vi "PathPlanner_TrajectoryState_Interpolate.vi"(9 "Time":dbl, 10 "end Val":T1={"AngularAcceleration"={"VALUE"=0.0, "COS"=1.0, "SIN"=0.0}, "PositionMeters"=0.0, "TrajectoryState"={"TimeSeconds"=0.0, "Velocity"=0.0, "Acceleration"=0.0, "POSE"={"TRANSLATION"={"X"=0.0, "Y"=0.0}, "ROTATION"={"VALUE"=0.0, "COS"=1.0, "SIN"=0.0}}, "Curvature"=0.0}, "AngularVelocity"={"VALUE"=0.0, "COS"=1.0, "SIN"=0.0}, "HolonomicRotation"={"VALUE"=0.0, "COS"=1.0, "SIN"=0.0}, "CurveRadius"=0.0, "DeltaPos"=0.0} {"HolonomicRotation"."SIN" format="%13.4f"; "HolonomicRotation"."COS" format="%13.4f"; "HolonomicRotation"."VALUE" format="%13.4f"; "AngularVelocity"."SIN" format="%13.4f"; "AngularVelocity"."COS" format="%13.4f"; "AngularVelocity"."VALUE" format="%13.4f"; "TrajectoryState"."POSE"."ROTATION"."SIN" format="%13.4f"; "TrajectoryState"."POSE"."ROTATION"."COS" format="%13.4f"; "TrajectoryState"."POSE"."ROTATION"."VALUE" format="%13.4f"; "TrajectoryState"."POSE"."TRANSLATION"."Y" format="%14.3f"; "TrajectoryState"."POSE"."TRANSLATION"."X" format="%14.3f"; "AngularAcceleration"."SIN" format="%13.4f"; "AngularAcceleration"."COS" format="%13.4f"; "AngularAcceleration"."VALUE" format="%13.4f"}, 11 "in PathPlannerState":T1={"AngularAcceleration"={"VALUE"=0.0, "COS"=1.0, "SIN"=0.0}, "PositionMeters"=0.0, "TrajectoryState"={"TimeSeconds"=0.0, "Velocity"=0.0, "Acceleration"=0.0, "POSE"={"TRANSLATION"={"X"=0.0, "Y"=0.0}, "ROTATION"={"VALUE"=0.0, "COS"=1.0, "SIN"=0.0}}, "Curvature"=0.0}, "AngularVelocity"={"VALUE"=0.0, "COS"=1.0, "SIN"=0.0}, "HolonomicRotation"={"VALUE"=0.0, "COS"=1.0, "SIN"=0.0}, "CurveRadius"=0.0, "DeltaPos"=0.0} {"HolonomicRotation"."SIN" format="%13.4f"; "HolonomicRotation"."COS" format="%13.4f"; "HolonomicRotation"."VALUE" format="%13.4f"; "AngularVelocity"."SIN" format="%13.4f"; "AngularVelocity"."COS" format="%13.4f"; "AngularVelocity"."VALUE" format="%13.4f"; "TrajectoryState"."POSE"."ROTATION"."SIN" format="%13.4f"; "TrajectoryState"."POSE"."ROTATION"."COS" format="%13.4f"; "TrajectoryState"."POSE"."ROTATION"."VALUE" format="%13.4f"; "TrajectoryState"."POSE"."TRANSLATION"."Y" format="%14.3f"; "TrajectoryState"."POSE"."TRANSLATION"."X" format="%14.3f"; "AngularAcceleration"."SIN" format="%13.4f"; "AngularAcceleration"."COS" format="%13.4f"; "AngularAcceleration"."VALUE" format="%13.4f"}) -> (3 "interpolated PathPlanner State":T1={"AngularAcceleration"={"VALUE"=0.0, "COS"=1.0, "SIN"=0.0}, "PositionMeters"=0.0, "TrajectoryState"={"TimeSeconds"=0.0, "Velocity"=0.0, "Acceleration"=0.0, "POSE"={"TRANSLATION"={"X"=0.0, "Y"=0.0}, "ROTATION"={"VALUE"=0.0, "COS"=1.0, "SIN"=0.0}}, "Curvature"=0.0}, "AngularVelocity"={"VALUE"=0.0, "COS"=1.0, "SIN"=0.0}, "HolonomicRotation"={"VALUE"=0.0, "COS"=1.0, "SIN"=0.0}, "CurveRadius"=0.0, "DeltaPos"=0.0} {"HolonomicRotation"."SIN" format="%13.4f"; "HolonomicRotation"."COS" format="%13.4f"; "HolonomicRotation"."VALUE" format="%13.4f"; "AngularVelocity"."SIN" format="%13.4f"; "AngularVelocity"."COS" format="%13.4f"; "AngularVelocity"."VALUE" format="%13.4f"; "TrajectoryState"."POSE"."ROTATION"."SIN" format="%13.4f"; "TrajectoryState"."POSE"."ROTATION"."COS" format="%13.4f"; "TrajectoryState"."POSE"."ROTATION"."VALUE" format="%13.4f"; "TrajectoryState"."POSE"."TRANSLATION"."Y" format="%14.3f"; "TrajectoryState"."POSE"."TRANSLATION"."X" format="%14.3f"; "AngularAcceleration"."SIN" format="%13.4f"; "AngularAcceleration"."COS" format="%13.4f"; "AngularAcceleration"."VALUE" format="%13.4f"})   [LabVIEW 2019, in "PathPlanner.lvlib"]
uses:
  PathPlanner.lvlib
  PathPlannerState.ctl
  <vilib>/Rock Robotics/WPI/ThirdParty/JAS_Junk/TrajLib/ROTATION2D.ctl
  <vilib>/Rock Robotics/WPI/ThirdParty/JAS_Junk/TrajLib/TRAJ_STATE.ctl
  <vilib>/Rock Robotics/WPI/ThirdParty/JAS_Junk/TrajLib/POSE2D.ctl
  <vilib>/Rock Robotics/WPI/ThirdParty/JAS_Junk/TrajLib/TRANSLATION2D.ctl
  <vilib>/Rock Robotics/WPI/ThirdParty/JAS_Junk/TrajLib/Trajectory_Library.lvlib
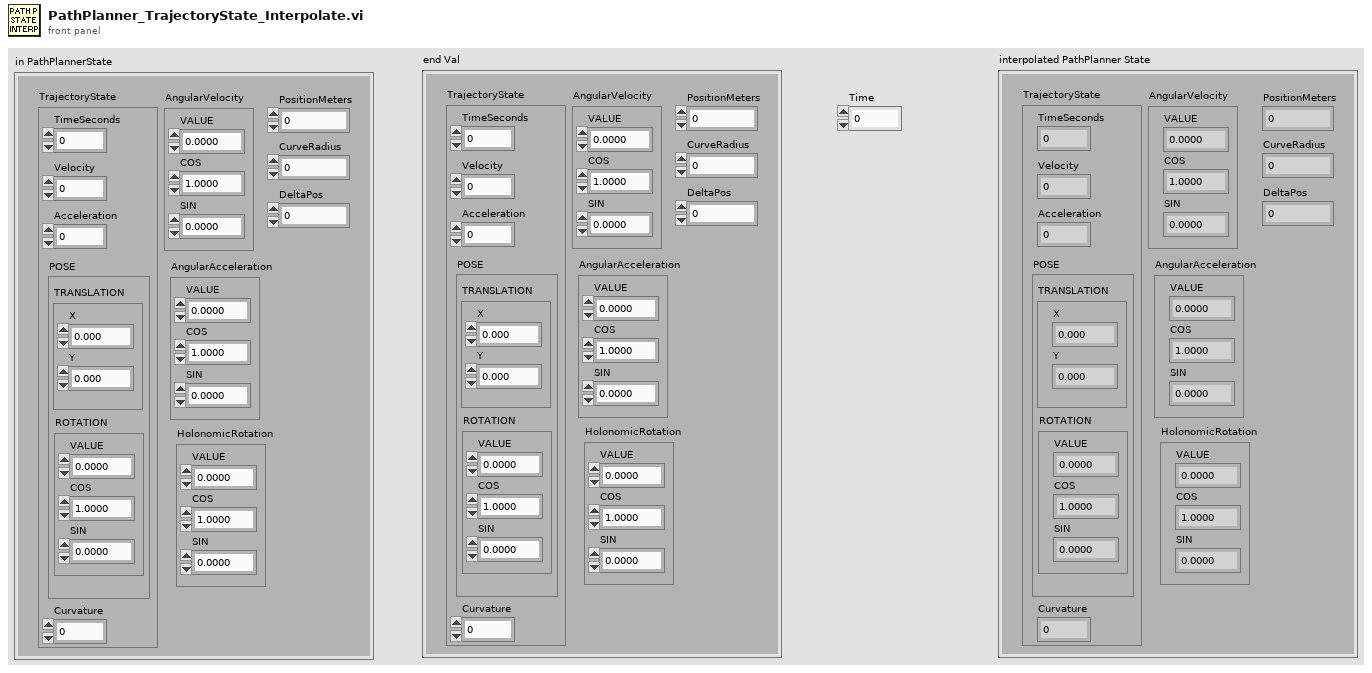
[diagram p1: front panel]
types:
  T1 = typedef "PathPlanner.lvlib/PathPlannerState.ctl" = cluster{"AngularAcceleration":T2, "PositionMeters":dbl, "TrajectoryState":T3, "AngularVelocity":T2, "HolonomicRotation":T2, "CurveRadius":dbl, "DeltaPos":dbl}
  T2 = typedef "Trajectory_Library.lvlib/ROTATION2D.ctl" = cluster{"VALUE":dbl, "COS":dbl, "SIN":dbl}
  T3 = typedef "Trajectory_Library.lvlib/TRAJ_STATE.ctl" = cluster{"TimeSeconds":dbl, "Velocity":dbl, "Acceleration":dbl, "POSE":T4, "Curvature":dbl}
  T4 = typedef "Trajectory_Library.lvlib/POSE2D.ctl" = cluster{"TRANSLATION":T5, "ROTATION":T2}
  T5 = typedef "Trajectory_Library.lvlib/TRANSLATION2D.ctl" = cluster{"X":dbl, "Y":dbl}
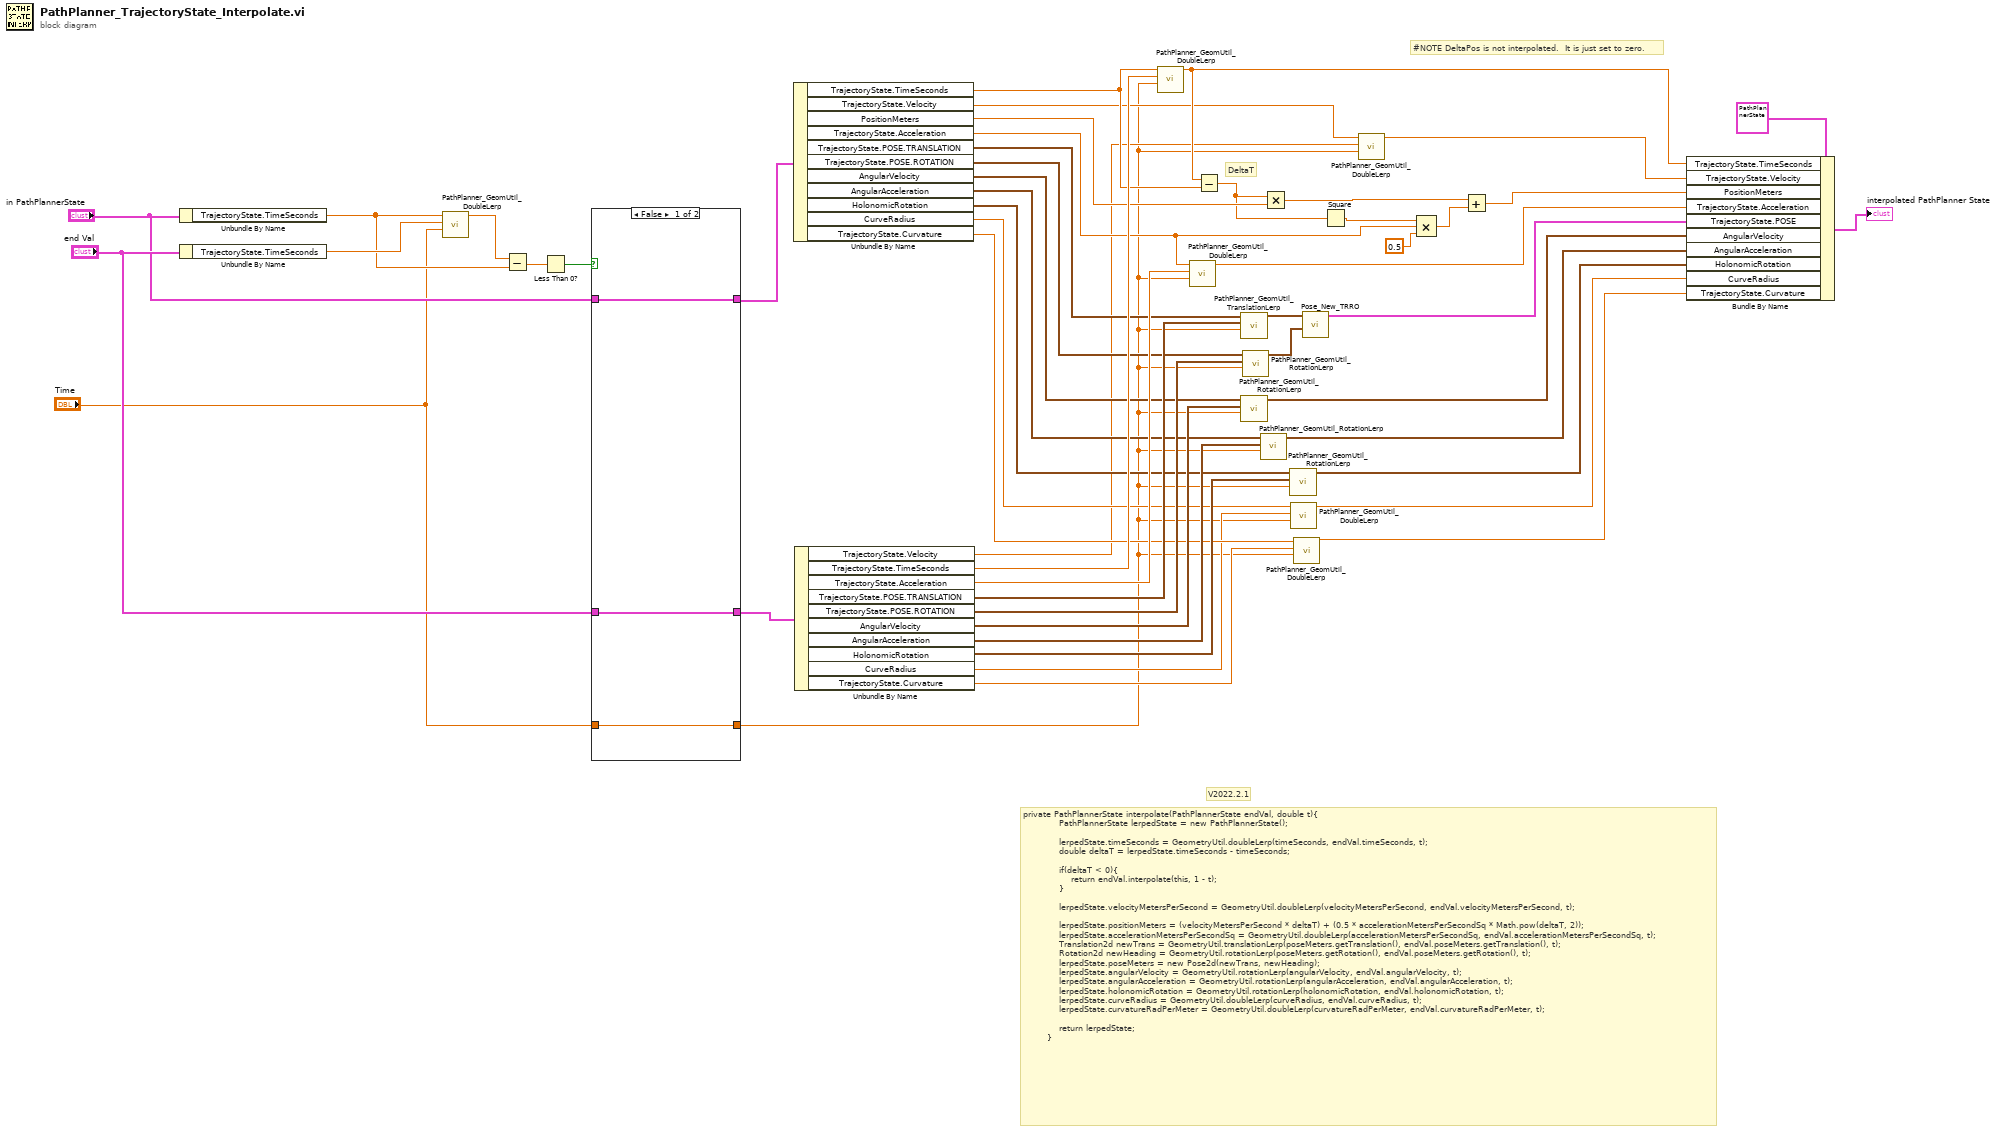
[diagram p0: block diagram]
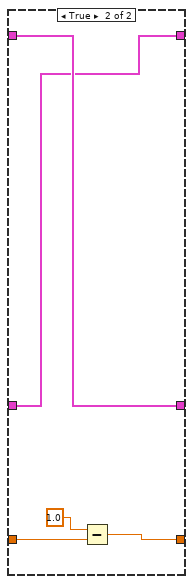
[diagram p2: hidden frame]
diagram:
  # "V2022.2.1"
  # "private PathPlannerState interpolate(PathPlannerState endVal, double t){\n            PathPlannerState lerpedState = new PathPlannerState();\n\n            lerpedState.timeSeconds = GeometryUtil.doubleLerp(timeSeconds, endVal.timeSeconds, t);\n            double deltaT = lerpedState.timeSeconds - timeSeconds;\n\n            if(deltaT < 0){\n                return endVal.interpolate(this, 1 - t);\n            }\n\n            lerpedState.velocityMetersPerSecond = GeometryUtil.doubleLerp(velocityMetersPerSecond, endVal.velocityMetersPerSecond, t);\n\n            lerpedState.positionMeters = (velocityMetersPerSecond * deltaT) + (0.5 * accelerationMetersPerSecondSq * Math.pow(deltaT, 2));\n            lerpedState.accelerationMetersPerSecondSq = GeometryUtil.doubleLerp(accelerationMetersPerSecondSq, endVal.accelerationMetersPerSecondSq, t);\n            Translation2d newTrans = GeometryUtil.translationLerp(poseMeters.getTranslation(), endVal.poseMeters.getTranslation(), t);\n            Rotation2d newHeading = GeometryUtil.rotationLerp(poseMeters.getRotation(), endVal.poseMeters.getRotation(), t);\n            lerpedState.poseMeters = new Pose2d(newTrans, newHeading);\n            lerpedState.angularVelocity = GeometryUtil.rotationLerp(angularVelocity, endVal.angularVelocity, t);\n            lerpedState.angularAcceleration = GeometryUtil.rotationLerp(angularAcceleration, endVal.angularAcceleration, t);\n            lerpedState.holonomicRotation = GeometryUtil.rotationLerp(holonomicRotation, endVal.holonomicRotation, t);\n            lerpedState.curveRadius = GeometryUtil.doubleLerp(curveRadius, endVal.curveRadius, t);\n            lerpedState.curvatureRadPerMeter = GeometryUtil.doubleLerp(curvatureRadPerMeter, endVal.curvatureRadPerMeter, t);\n\n            return lerpedState;\n        }"
  # "#NOTE DeltaPos is not interpolated.  It is just set to zero."
  # "DeltaT"
  n1 = Unbundle By Name("in PathPlannerState") -> ("TrajectoryState.TimeSeconds"=w47:dbl)
  n2 = Unbundle By Name("end Val") -> ("TrajectoryState.TimeSeconds"=w49:dbl)
  n3 = call "PathPlanner_GeomUtil_DoubleLerp.vi"("T"="Time", "EndVal"=w49, "StartVal"=w47) -> ("Lerp"=w48:dbl)  [unwired: 8 in]
  n4 = Subtract(x=w48, y=w47) -> (x-y=w46:dbl)
  n5 = Less Than 0?(x=w46) -> (x < 0?=w45:bool)
  n6 = case shown="False" w45 {
    tunnel: "end Val" -> [w54 w58]
    tunnel: [w54 w59] -> w40
    tunnel: "in PathPlannerState" -> [w53 w59]
    tunnel: [w53 w58] -> w41
    tunnel: [w52 w55] -> w1
    tunnel: "Time" -> [w52 w56]
    frame False {
    }
    frame True {
      n7 = Subtract(x=1.0, y=w56) -> (x-y=w55:dbl)
    }
  }
  n8 = Unbundle By Name(w41) -> ("TrajectoryState.TimeSeconds"=w37:dbl, "TrajectoryState.Velocity"=w3:dbl, "PositionMeters"=w36:dbl, "TrajectoryState.Acceleration"=w29:dbl, "TrajectoryState.POSE.TRANSLATION"=w26:T5, "TrajectoryState.POSE.ROTATION"=w24:T2, "AngularVelocity"=w19:T2, "AngularAcceleration"=w16:T2, "HolonomicRotation"=w13:T2, "CurveRadius"=w10:dbl, "TrajectoryState.Curvature"=w9:dbl)
  n9 = Unbundle By Name(w40) -> ("TrajectoryState.Velocity"=w2:dbl, "TrajectoryState.TimeSeconds"=w39:dbl, "TrajectoryState.Acceleration"=w28:dbl, "TrajectoryState.POSE.TRANSLATION"=w25:T5, "TrajectoryState.POSE.ROTATION"=w23:T2, "AngularVelocity"=w18:T2, "AngularAcceleration"=w15:T2, "HolonomicRotation"=w12:T2, "CurveRadius"=w8:dbl, "TrajectoryState.Curvature"=w7:dbl)
  n10 = call "PathPlanner_GeomUtil_DoubleLerp.vi"("T"=w1, "EndVal"=w39, "StartVal"=w37) -> ("Lerp"=w38:dbl)  [unwired: 8 in]
  n11 = call "PathPlanner_GeomUtil_DoubleLerp.vi"("T"=w1, "EndVal"=w28, "StartVal"=w29) -> ("Lerp"=w27:dbl)  [unwired: 8 in]
  n12 = Subtract(x=w38, y=w37) -> (x-y=w30:dbl)
  n13 = call "PathPlanner_GeomUtil_TranslationLerp.vi"("T"=w1, "EndVal"=w25, "StartVal"=w26) -> ("Lerp"=w22:T5)  [unwired: 8 in]
  n14 = call "PathPlanner_GeomUtil_RotationLerp.vi"("T"=w1, "EndVal"=w18, "StartVal"=w19) -> ("Lerp"=w17:T2)  [unwired: 8 in]
  n15 = call "PathPlanner_GeomUtil_RotationLerp.vi"("T"=w1, "EndVal"=w23, "StartVal"=w24) -> ("Lerp"=w21:T2)  [unwired: 8 in]
  n16 = call "PathPlanner_GeomUtil_RotationLerp.vi"("T"=w1, "EndVal"=w15, "StartVal"=w16) -> ("Lerp"=w14:T2)  [unwired: 8 in]
  n17 = Multiply(x=w30, y=w36) -> (x*y=w34:dbl)
  n18 = call "PathPlanner_GeomUtil_RotationLerp.vi"("T"=w1, "EndVal"=w12, "StartVal"=w13) -> ("Lerp"=w11:T2)  [unwired: 8 in]
  n19 = call "PathPlanner_GeomUtil_DoubleLerp.vi"("T"=w1, "EndVal"=w8, "StartVal"=w10) -> ("Lerp"=w6:dbl)  [unwired: 8 in]
  n20 = call "PathPlanner_GeomUtil_DoubleLerp.vi"("T"=w1, "EndVal"=w7, "StartVal"=w9) -> ("Lerp"=w5:dbl)  [unwired: 8 in]
  n21 = call <vilib>:"Pose_New_TRRO.vi"("ROTATION"=w21, "TRANSLATION"=w22) -> ("outPOSE"=w20:T4)  [unwired: 9 in]
  n22 = Square(x=w30) -> (x^2=w31:dbl)
  n23 = call "PathPlanner_GeomUtil_DoubleLerp.vi"("T"=w1, "EndVal"=w2, "StartVal"=w3) -> ("Lerp"=w4:dbl)  [unwired: 8 in]
  n24 = Compound Arithmetic op=MULTIPLY(w31, w29, 0.5 ("value")) -> (w33:dbl)
  n25 = Add(x=w34, y=w33) -> (x+y=w35:dbl)
  n26 = Bundle By Name(cluster=T1 {"AngularAcceleration"={"VALUE"=0.0, "COS"=1.0, "SIN"=0.0}, "PositionMeters"=0.0, "TrajectoryState"={"TimeSeconds"=0.0, "Velocity"=0.0, "Acceleration"=0.0, "POSE"={"TRANSLATION"={"X"=0.0, "Y"=0.0}, "ROTATION"={"VALUE"=0.0, "COS"=1.0, "SIN"=0.0}}, "Curvature"=0.0}, "AngularVelocity"={"VALUE"=0.0, "COS"=1.0, "SIN"=0.0}, "HolonomicRotation"={"VALUE"=0.0, "COS"=1.0, "SIN"=0.0}, "CurveRadius"=0.0, "DeltaPos"=0.0} ("PathPlannerState"), "TrajectoryState.TimeSeconds"=w38, "TrajectoryState.Velocity"=w4, "PositionMeters"=w35, "TrajectoryState.Acceleration"=w27, "TrajectoryState.POSE"=w20, "AngularVelocity"=w17, "AngularAcceleration"=w14, "HolonomicRotation"=w11, "CurveRadius"=w6, "TrajectoryState.Curvature"=w5) -> (→"interpolated PathPlanner State":T1)
